vi "Proceed.vi"(7 "component is ready (Y)":bool=TRUE, 8 "error in (no error)":errorcluster, 10 "ProceedMessage":refnum<class "ProceedMessage.lvclass">, 11 "ImageStack in":refnum<class "ImageStack.lvclass">) -> (0 "error out":errorcluster, 2 "all observers are ready?":bool, 3 "ImageStack out":refnum<class "ImageStack.lvclass">)   [LabVIEW 2012, in "ImageStack.lvclass"]
uses:
  ImageStack.lvclass
  <vilib>/Distrio/Murmex/ProceedMessage/ProceedMessage.lvclass
  ImageStack.lvclass/ImageStack.ctl
  <vilib>/Distrio/Murmex/Murmex/Murmex.lvclass
  <vilib>/Distrio/Murmex/Message/Message.lvclass
panel:
  # "This method is called when the PROCEED\ntrigger is sent. \n\nOverride this method when your component needs to\nrespond to this trigger. \n\nCall parent for proper implementation"
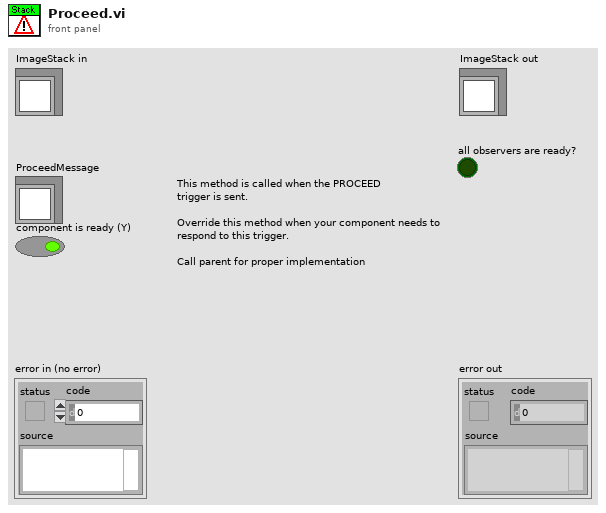
[diagram p1: front panel]
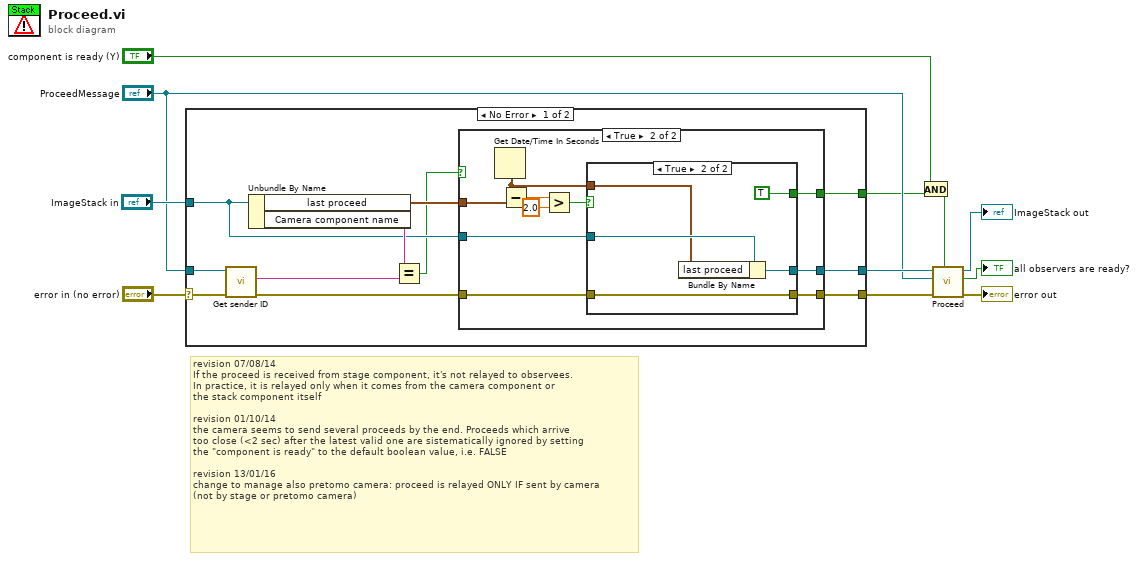
[diagram p0: block diagram]
diagram:
  # "revision 07/08/14\nIf the proceed is received from stage component, it's not relayed to observees.\nIn practice, it is relayed only when it comes from the camera component or \nthe stack component itself\n\nrevision 01/10/14\nthe camera seems to send several proceeds by the end. Proceeds which arrive\ntoo close (<2 sec) after the latest valid one are sistematically ignored by setting\nthe \"component is ready\" to the default boolean value, i.e. FALSE\n\nrevision 13/01/16\nchange to manage also pretomo camera: proceed is relayed ONLY IF sent by camera\n(not by stage or pretomo camera)"
  n1 = case shown="No Error" "error in (no error)" {
    selector: "error in (no error)" -> [w21 w42]
    tunnel: "ImageStack in" -> [w16 w43]
    tunnel: [w13 w42] -> w6
    tunnel: [w14 w43] -> w5
    tunnel: "ProceedMessage" -> [w22 _]
    tunnel: [w15 _] -> w3
    frame No Error {
      n2 = call <vilib>:"Get sender ID.vi"("error in (no error)"=w21, "Message in"=w22) -> ("error out"=w18:errorcluster, "sender"=w20:string)  [unwired: 7 in, 1 out]
      n3 = Unbundle By Name(w16) -> ("last proceed"=w17:timestamp, "Camera component name"=w19:string)
      n4 = Equal?(x=w19, y=w20) -> (x = y?=w12:bool)
      n5 = case shown="True" w12 {
        tunnel: w18 -> [w23 w25]
        tunnel: w17 -> [_ w34]
        tunnel: w16 -> [w24 w30]
        tunnel: [_ w29] -> w15
        tunnel: [w24 w28] -> w14
        tunnel: [w23 w26] -> w13
        frame False {
        }
        frame True {
          n6 = Get Date/Time In Seconds() -> (seconds since 1Jan1904=w27:timestamp)
          n7 = Subtract(x=w27, y=w34) -> (x-y=w33:dbl)
          n8 = Greater?(x=w33, y=2.0) -> (0:w31:bool)
          n9 = case shown="True" w31 {
            tunnel: w30 -> [w36 w40]
            tunnel: [_ TRUE] -> w29
            tunnel: [w36 w39] -> w28
            tunnel: w27 -> [_ w38]
            tunnel: [w35 w37] -> w26
            tunnel: w25 -> [w35 w37]
            frame False {
            }
            frame True {
              n10 = Bundle By Name(cluster=w40, "last proceed"=w38) -> (w39:refnum<class "ImageStack.lvclass">)
            }
          }
        }
      }
    }
    frame Error {
    }
  }
  n11 = And(x="component is ready (Y)", y=w3) -> (x .and. y?=w1:bool)
  n12 = call-parent "Proceed.vi"("component is ready (Y)"=w1, "error in (no error)"=w6, "ProceedMessage"="ProceedMessage", "Murmex in"=w5) -> ("error out"=→"error out":errorcluster, "all observers are ready?"=→"all observers are ready?":bool, "Murmex out"=→"ImageStack out":refnum<class "ImageStack.lvclass">)  [unwired: 5 in]
